vi "Process Tovey Data.vi"(8 "error in (no error)":errorcluster, 11 "Model in":refnum<class "Model.lvclass">) -> (0 "error out":errorcluster, 3 "Model out":refnum<class "Model.lvclass">)   [LabVIEW 2016, in "Model.lvclass"]
uses:
  Model.lvclass
  Model.lvclass/Model.ctl
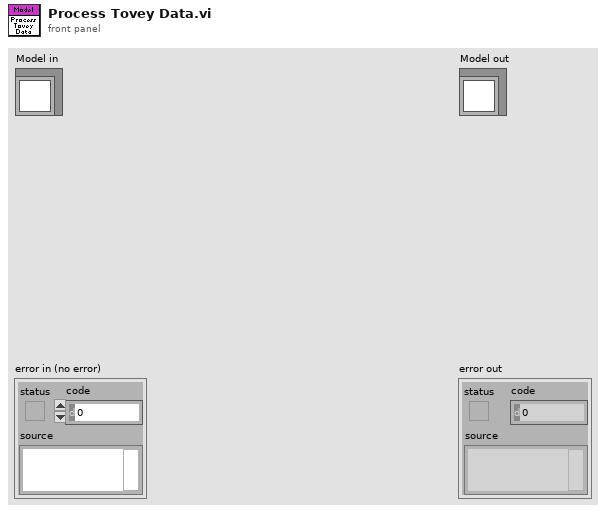
[diagram p1: front panel]
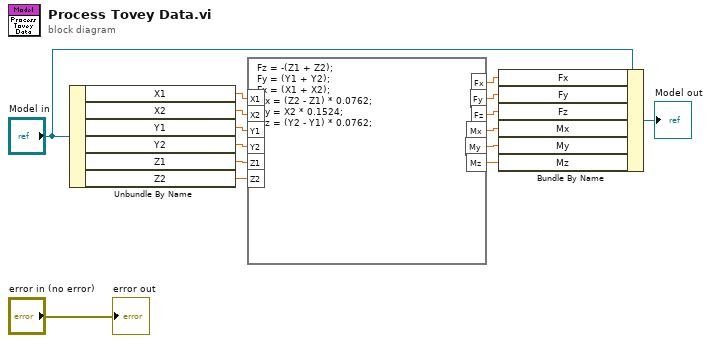
[diagram p0: block diagram]
diagram:
  n1 = Unbundle By Name("Model in") -> ("X1"=w13:dbl, "X2"=w12:dbl, "Y1"=w11:dbl, "Y2"=w10:dbl, "Z1"=w9:dbl, "Z2"=w8:dbl)
  n2 = formula code="Fz = -(Z1 + Z2);\nFy = (Y1 + Y2);\nFx = (X1 + X2);\nMx = (Z2 - Z1) * 0.0762;\nMy = X2 * 0.1524;\nMz = (Y2 - Y1) * 0.0762;"("X1"=w13, "X2"=w12, "Y1"=w11, "Y2"=w10, "Z1"=w9, "Z2"=w8) -> ("Fx"=w7:dbl, "Fy"=w6:dbl, "Fz"=w5:dbl, "Mx"=w4:dbl, "My"=w3:dbl, "Mz"=w2:dbl)
  n3 = Bundle By Name(cluster="Model in", "Fx"=w7, "Fy"=w6, "Fz"=w5, "Mx"=w4, "My"=w3, "Mz"=w2) -> (→"Model out":refnum<class "Model.lvclass">)
  "error out" <- "error in (no error)"
